vi "Fetch Background Measurements (Energy).vi"(0 "VISA resource name":refnum<visa-resource-name>, 11 "error in (no error)":errorcluster) -> (4 "VISA resource name out":refnum<visa-resource-name>, 6 "Energy Measurements":T1, 15 "error out":errorcluster)   [LabVIEW 2012, in "NH Research Regenerative Test Series.lvlib"]
doc: "Returns the most recent energy measurements that are always being made by the hardware in the background (except while a waveform capture is being made)."
uses:
  <instrlib>/NH Research Regenerative Test Series/NH Research Regenerative Test Series.lvlib
  <instrlib>/NH Research Regenerative Test Series/Public/Data/Energy Measurements.ctl
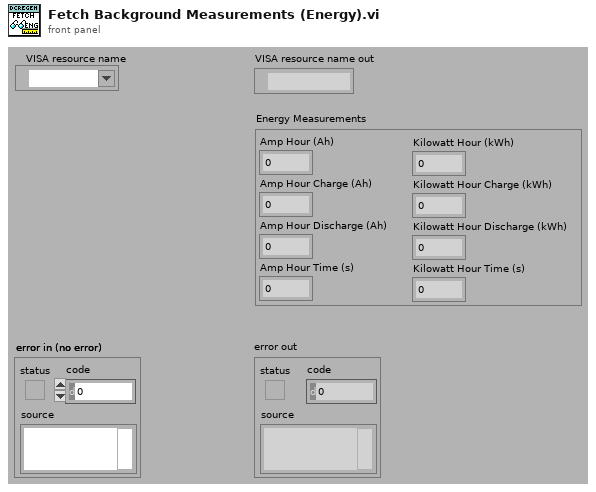
[diagram p1: front panel]
types:
  T1 = typedef "NH Research Regenerative Test Series.lvlib/Energy Measurements.ctl" = cluster{"Amp Hour (Ah)":dbl, "Amp Hour Charge (Ah)":dbl, "Amp Hour Discharge (Ah)":dbl, "Amp Hour Time (s)":dbl, "Kilowatt Hour (kWh)":dbl, "Kilowatt Hour Charge (kWh)":dbl, "Kilowatt Hour Discharge (kWh)":dbl, "Kilowatt Hour Time (s)":dbl}
  T2 = cluster{"[0]":dbl, "[1]":dbl, "[2]":dbl, "[3]":dbl, "[4]":dbl, "[5]":dbl, "[6]":dbl, "[7]":dbl}
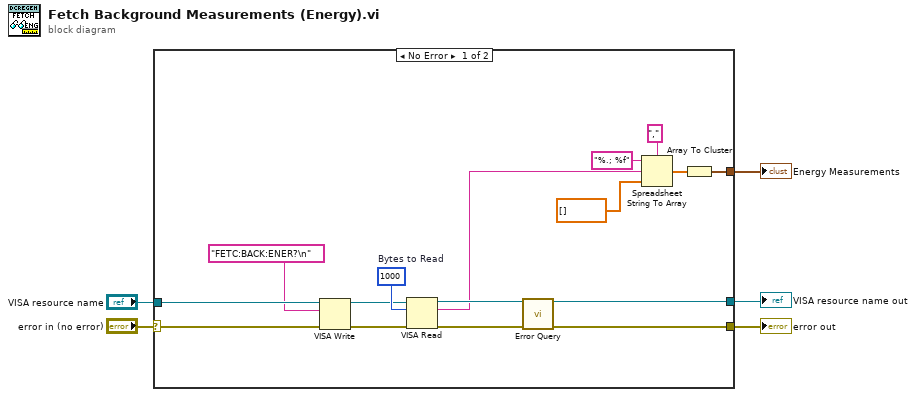
[diagram p0: block diagram]
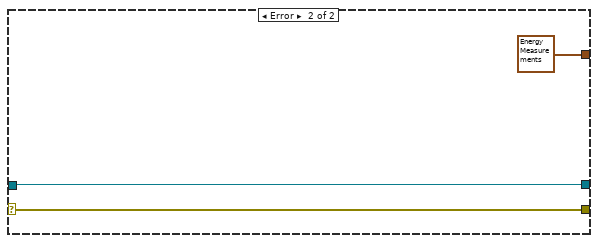
[diagram p2: hidden frame]
diagram:
  n1 = case shown="No Error" "error in (no error)" {
    selector: "error in (no error)" -> [w10 w24]
    tunnel: [w17 w24] -> w4
    tunnel: [w20 w23] -> w2
    tunnel: "VISA resource name" -> [w9 w23]
    tunnel: [w12 T1 {"Amp Hour (Ah)"=nan, "Amp Hour Charge (Ah)"=nan, "Amp Hour Discharge (Ah)"=nan, "Amp Hour Time (s)"=nan, "Kilowatt Hour (kWh)"=nan, "Kilowatt Hour Charge (kWh)"=nan, "Kilowatt Hour Discharge (kWh)"=nan, "Kilowatt Hour Time (s)"=nan}] -> w1
    frame No Error {
      w21 = u32 1000  # Bytes to Read
      n2 = VISA Write(VISA resource name=w9, write buffer="FETC:BACK:ENER?\n" ("Command"), error in (no error)=w10) -> (VISA resource name out=w8:refnum<visa-resource-name>, error out=w7:errorcluster)  [unwired: 1 out]
      n3 = VISA Read(VISA resource name=w8, byte count=w21, error in (no error)=w7) -> (VISA resource name out=w19:refnum<visa-resource-name>, read buffer=w11:string, error out=w18:errorcluster)  [unwired: 1 out]
      n4 = call <instrlib>:"Error Query.vi"("VISA resource name"=w19, "error in (no error)"=w18) -> ("VISA resource name out"=w20:refnum<visa-resource-name>, "error out"=w17:errorcluster)  [unwired: 10 in, 2 out]
      n5 = Spreadsheet String To Array(delimiter (Tab)=",", format string="%.; %f", spreadsheet string=w11, array type (2D Dbl)=dbl[] []) -> (array=w13:dbl[])
      n6 = Array To Cluster(array=w13) -> (cluster=w12:T2)
    }
    frame Error {
    }
  }
  "error out" <- w4
  "VISA resource name out" <- w2
  "Energy Measurements" <- w1
